vi "remove button action.vi"(6 "user event":T1, 7 "channel list":refnum<vi>, 8 "error in":errorcluster, 9 "channel":i32, 10 "Engine Configuration in":refnum<class "engine configuration.lvclass">, 11 "EIP Tags Configuration in":refnum<class "EIP Tags Configuration.lvclass">) -> (0 "error out":errorcluster, 2 "Engine Configuration out":refnum<class "engine configuration.lvclass">, 3 "EIP Tags Configuration out":refnum<class "EIP Tags Configuration.lvclass">)   [LabVIEW 2013, in "EIP Tags editor node.lvclass"]
uses:
  EIP Tags editor node.lvclass
  <vilib>/NI/Configuration Framework/Controls/EventCluster.ctl
  <vilib>/NI/Configuration Framework/NISE_CEF_TreeControl.lvlib
  <vilib>/NI/Module Execution Interface/Engine Configuration/engine configuration.lvclass
  configuration/EIP Tags Configuration.lvclass
  <vilib>/NI/Configuration Framework/serializable configuration/NISE_CEF_serializable configuration.lvclass
  <vilib>/NI/Configuration Framework/Node/UserEventRef.ctl
  <vilib>/NI/Configuration Framework/Node/NISE_CEF_Node.lvclass
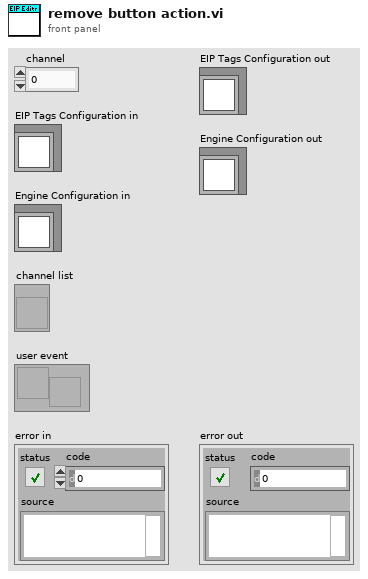
[diagram p1: front panel]
types:
  T1 = typedef "NISE_CEF_Node.lvclass/UserEventRef.ctl" = refnum<user-event>
  T2 = typedef "EIP Tags editor node.lvclass/table line.ctl" = cluster{"eip channel":refnum<class "EIP Tags Channel.lvclass">, "tag name":string}
  T3 = typedef "NISE_CEF_TreeControl.lvlib/EventCluster.ctl" = cluster{"command":string, "data":string}
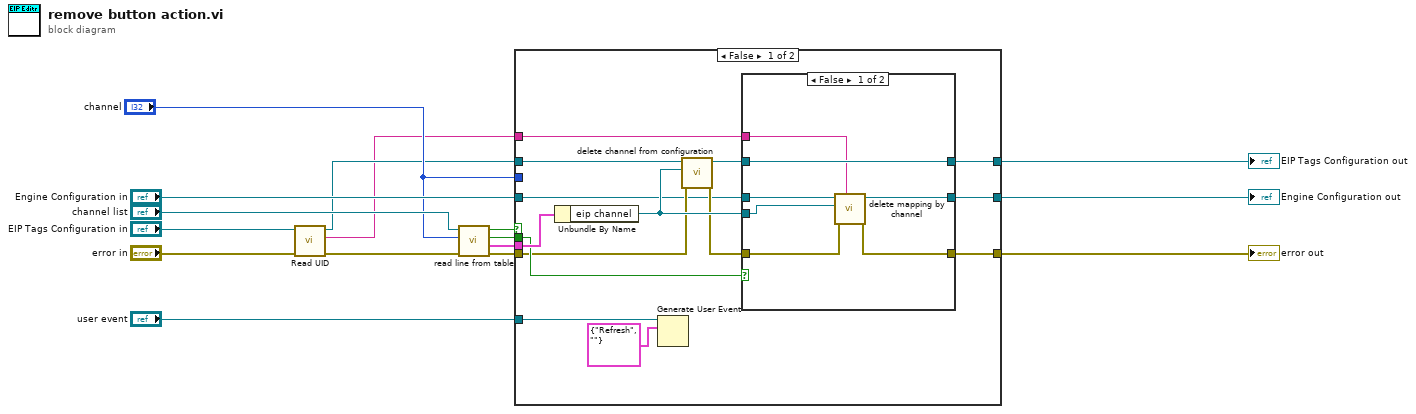
[diagram p0: block diagram]
diagram:
  n1 = call <vilib>:"Read UID.vi"("error in"="error in", "configuration in"="EIP Tags Configuration in") -> ("error out"=w4:errorcluster, "instance id"=w1:string, "configuration out"=w2:refnum<class "EIP Tags Configuration.lvclass">)  [unwired: 7 in]
  n2 = call "read line from table.vi"("error in"=w4, "line number"="channel", "channels table"="channel list") -> ("error out"=w11:errorcluster, "line"=w7:T2, "empty tag?"=w10:bool, "empty channel?"=w9:bool)  [unwired: 5 in]
  n3 = case shown="False" w9 {
    tunnel: [w20 w42] -> w5
    tunnel: "channel" -> [_ _]
    tunnel: w7 -> [w30 _]
    tunnel: w2 -> [w28 w41]
    tunnel: "Engine Configuration in" -> [w23 w43]
    tunnel: w10 -> [w29 _]
    tunnel: w11 -> [w26 w42]
    tunnel: [w22 w43] -> w15
    tunnel: [w21 w41] -> w14
    tunnel: "user event" -> [w18 _]
    tunnel: w1 -> [w17 _]
    frame False {
      n4 = Unbundle By Name(w30) -> ("eip channel"=w27:refnum<class "EIP Tags Channel.lvclass">)
      n5 = Generate User Event(user event=w18, event data cluster=T3 {"command"="Refresh", "data"=""} ("event data")) -> ()  [unwired: 2 in, 2 out]
      n6 = call "delete channel from configuration.vi"("error in"=w26, "TBM channel in"=w27, "EthernetIP configuration in"=w28) -> ("error out"=w24:errorcluster, "EthernetIP configuration out"=w25:refnum<class "EIP Tags Configuration.lvclass">)  [unwired: 7 in]
      n7 = case shown="False" w29 {
        tunnel: w27 -> [w36 _]
        tunnel: w25 -> [w32 w38]
        tunnel: w24 -> [w35 w39]
        tunnel: w23 -> [w37 w40]
        tunnel: [w34 w40] -> w22
        tunnel: [w33 w39] -> w20
        tunnel: [w32 w38] -> w21
        tunnel: w17 -> [w31 _]
        frame False {
          n8 = call <vilib>:"delete mapping by channel.vi"("owner ID"=w31, "error in"=w35, "channel"=w36, "engine configuration in"=w37) -> ("error out"=w33:errorcluster, "engine configuration out"=w34:refnum<class "engine configuration.lvclass">)  [unwired: 6 in]
        }
        frame True {
        }
      }
    }
    frame True {
    }
  }
  "Engine Configuration out" <- w15
  "EIP Tags Configuration out" <- w14
  "error out" <- w5
